vi "VI, Grow Panel Size.vi"(4 "Y margin (8)":i16=8, 5 "X margin (8)":i16=8, 6 "error in":errorcluster, 9 "VI ref":refnum<vi>) -> (0 "error out":errorcluster, 3 "VI ref dup":refnum<vi>)   [LabVIEW 2010]
doc: "This function increases the panel width and height to display all controls on the panel."
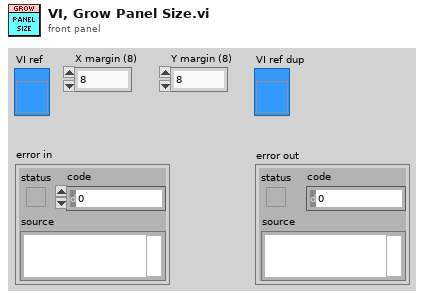
[diagram p1: front panel]
types:
  T1 = typedef "LVRectTypeDef.ctl" = cluster{"left":i16, "top":i16, "right":i16, "bottom":i16}
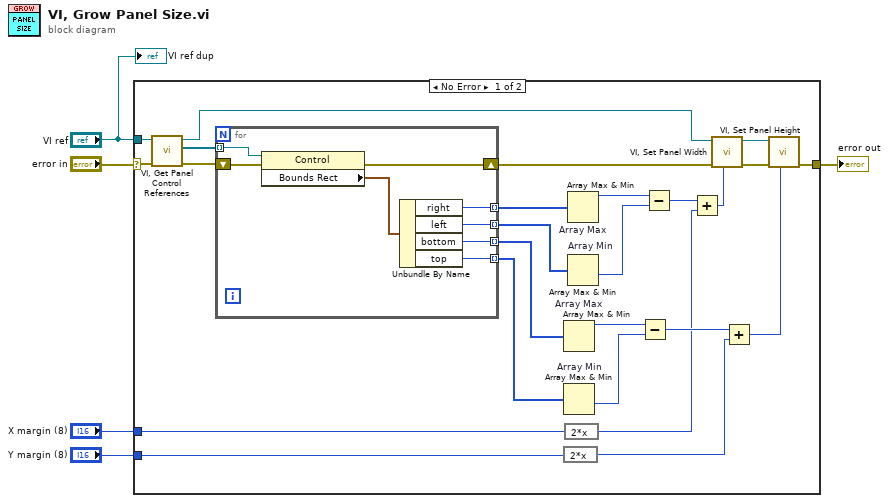
[diagram p0: block diagram]
diagram:
  n1 = case shown="No Error" "error in" {
    selector: "error in" -> [w23 w39]
    tunnel: "VI ref" -> [w22 _]
    tunnel: [w10 w39] -> w3
    tunnel: "X margin (8)" -> [w24 _]
    tunnel: "Y margin (8)" -> [w12 _]
    frame No Error {
      n2 = call "VI, Get Panel Control References.vi"("error in"=w23, "VI ref"=w22) -> ("error out"=w21:errorcluster, "Ctl refnum array"=w19:refnum<vi>[], "VI ref dup"=w20:refnum<vi>)  [unwired: 5 in]
      n3 = for {
        tunnel: [w37] -> w30 mode=indexing
        tunnel: [w36] -> w18 mode=indexing
        shift-right: [w35] -> w27
        shift-left: w21 -> [w34]
        tunnel: w19 -> [w33] mode=indexing
        tunnel: [w32] -> w14 mode=indexing
        tunnel: [w31] -> w13 mode=indexing
        n4 = property class="Control"(reference=w33, error in=w34) -> (error out=w35:errorcluster, "Bounds Rect"=w38:T1)  [unwired: 1 out]
        n5 = Unbundle By Name(w38) -> ("right"=w37:i16, "left"=w36:i16, "bottom"=w32:i16, "top"=w31:i16)
      }
      n6 = Array Max & Min "Array Max"(array=w14) -> (max value=w15:i16)  [unwired: 3 out]
      n7 = Array Max & Min "Array Min"(array=w13) -> (min value=w16:i16)  [unwired: 3 out]
      n8 = expression code="2*x"(w12) -> (w6:i16)
      n9 = expression code="2*x"(w24) -> (w7:i16)
      n10 = Array Max & Min "Array Max"(array=w30) -> (max value=w29:i16)  [unwired: 3 out]
      n11 = Array Max & Min "Array Min"(array=w18) -> (min value=w28:i16)  [unwired: 3 out]
      n12 = Subtract(x=w15, y=w16) -> (x-y=w17:i16)
      n13 = Subtract(x=w29, y=w28) -> (x-y=w26:i16)
      n14 = Add(x=w26, y=w7) -> (x+y=w25:i16)
      n15 = call "VI, Set Panel Width.vi"("width"=w25, "error in"=w27, "VI ref"=w20) -> ("error out"=w11:errorcluster, "VI ref dup"=w9:refnum<vi>)  [unwired: 5 in]
      n16 = Add(x=w17, y=w6) -> (x+y=w8:i16)
      n17 = call "VI, Set Panel Height.vi"("height"=w8, "error in"=w11, "VI ref"=w9) -> ("error out"=w10:errorcluster)  [unwired: 5 in, 1 out]
    }
    frame Error {
    }
  }
  "error out" <- w3
  "VI ref dup" <- "VI ref"
